vi "dfd_nMAC_CircSubONEwEn.vi"(1 "len":fxp<+,16,16>, 2 "idxIn":fxp<+,16,16>, 3 "Enable":bool) -> (6 "wrap?":bool, 7 "idxOut":fxp<+,16,16>)   [LabVIEW 2017]
doc: "wrap? is cleared if Enable==False."
uses:
  <vilib>/rvi/FXPMathLib/basic elements/FxpAddSub/XNode/nifxpmath_AddSub.xnode
  <vilib>/rvi/FXPMathLib/sim/FxpSim.dll
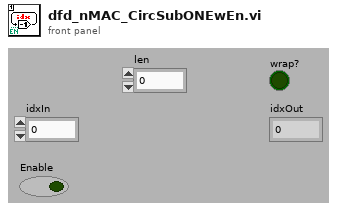
[diagram p1: front panel]
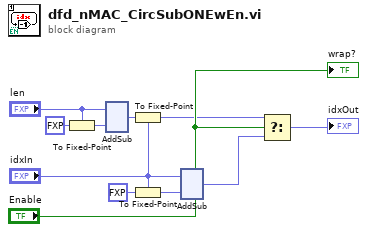
[diagram p0: block diagram]
diagram:
  n1 = To Fixed-Point(fixed-point type="len", number=fxp<+,1,1> 1.0 ("y")) -> (fixed-point=w5:fxp<+,16,16>)
  n2 = xnode "AddSub"("x"="len", "y"=w5) -> ("s"=w7:fxp<+,16,16>)  [unwired: 1 out]
  n3 = To Fixed-Point(fixed-point type="idxIn", number=w7) -> (fixed-point=w4:fxp<+,16,16>)
  n4 = To Fixed-Point(fixed-point type="idxIn", number=fxp<+,1,1> 0.0 ("step")) -> (fixed-point=w3:fxp<+,16,16>)
  n5 = xnode "AddSub"("x"="idxIn", "y"=w3, "borrow-in"="Enable") -> ("s"=w11:fxp<+,16,16>, "borrow-out"=w10:bool)
  "wrap?" <- w10
  n6 = Select(t=w4, s=w10, f=w11) -> (s? t:f=→"idxOut":fxp<+,16,16>)
